vi "MTExam.vi"() -> ()   [LabVIEW 2016]
uses:
  VIs/uPythonX/uPythonX.xctl
panel:
  in  "WiFi":T1(xcontrol)={"VISA Refnum in"="ASRL44::INSTR", "Python Code"="import machine, network, ubinascii, ujson, urequests, utime,gc\nfrom pyb import LED\n\nWiFi = network.WLAN()\n\nmac = ubinascii.hexlify(network.WLAN().config(\"mac\"),\":\").decode()\nprint(\"MAC address: \" + mac)\ndef connect():\n     if not WiFi.isconnected():\n          print (\"Connecting ..\")\n          WiFi.active(True)\n          WiFi.connect(\"Rogers\",\"s0meth1ng\")\n          i=0\n          while i < 25 and not WiFi.isconnected():\n               utime.sleep_ms(200)\n               i=i+1\n          if WiFi.isconnected():\n               print (\"Connection succeeded\")\n          else:\n               print (\"Connection failed\")     \n     return WiFi.isconnected()\n\n# Systemlink\nKey = \"dYy-vDU9TXxDCy2QG3jO4J0s1-QUyYs6sO1xPd1oKQ\"\n\nurlBase = \"https://api.systemlinkcloud.com/nitag/v2/tags/\"\n\nheaders = {\"Accept\":\"application/json\",\"x-ni-api-key\":Key}\n\ndef Put(tag,type,value):\n     urlTag = urlBase + tag\n     urlValue = urlBase + tag + \"/values/current\"\n     propName={\"type\":type,\"path\":tag}\n     propValue = {\"value\":{\"type\":type,\"value\":value}}\n     #  assume that the tag is already created  -      urequests.put(urlTag,headers=headers,json=propName).text\n     try:\n          response = urequests.put(urlValue,headers=headers,json=propValue)\n          print(response.text)\n          response.close()\n     except:\n          print('error')\n\ndef Get(tag):\n     urlValue = urlBase + tag + \"/values/current\"\n     try:\n          response = urequests.get(urlValue,headers=headers)\n          value = response.text\n          response.close()\n          print(value)\n          data = ujson.loads(value)\n          result = data.get(\"value\").get(\"value\")\n     except:\n          print('error')\n          result = 'error'\n     return result\n\nprint (\"WiFi: \",connect())\nPut('EV3','U_INT64','3')\nGet('EV3')\nGet('msec')\nPut('msec','INT',100)\nled = LED(1) # 1=red, 2=green, 3=blue\n\ni=0\nold = utime.ticks_ms()\nwhile True:\n     Put('EV3','U_INT64',str(i))\n     new = utime.ticks_ms()\n     Put('msec','INT',str(new-old))\n     old = new\n     i= i + 1\n     print(i)\n     led.toggle()\n     utime.sleep_ms(20)\n     gc.collect()\n\n\n\n\n\n\n"}
  in  "PyBoard - Tacho":T1(xcontrol)={"VISA Refnum in"="ASRL44::INSTR", "Python Code"="# From https://github.com/peterhinch/micropython-samples/blob/master/encoders/encoder.py\n\nfrom pyb import Pin\nimport utime\nfrom machine import UART\n\nuart = UART(3)  #TX = Y9\nuart.init(9600, bits=8, parity=None, stop=1)\n\nclass Encoder(object):\n     def __init__(self, pin_x, pin_y, reverse, scale):\n          self.reverse = reverse\n          self.scale = scale\n          self.forward = True\n          self.pin_x = pin_x\n          self.pin_y = pin_y\n          self._pos = 0\n          self.x_interrupt = pyb.ExtInt(pin_x, pyb.ExtInt.IRQ_RISING_FALLING, pyb.Pin.PULL_NONE, self.x_callback)\n          self.y_interrupt = pyb.ExtInt(pin_y, pyb.ExtInt.IRQ_RISING_FALLING, pyb.Pin.PULL_NONE, self.y_callback)\n\n     def x_callback(self, line):\n          self.forward = self.pin_x.value() ^ self.pin_y.value() ^ self.reverse\n          self._pos += 1 if self.forward else -1\n\n     def y_callback(self, line):\n          self.forward = self.pin_x.value() ^ self.pin_y.value() ^ self.reverse ^ 1\n          self._pos += 1 if self.forward else -1\n\n     @property\n     def position(self):\n          return self._pos*self.scale\n\n     def reset(self):\n          self._pos = 0\n\npin1 = Pin('Y4', Pin.IN)\npin2 = Pin('Y3', Pin.IN)\n\ne=Encoder(pin1,pin2,False,0.5)\ne.reset()\nwhile True:\n     value = e.position\n     sent = uart.write('%d\\n' % int(value/10))\n     print(value)\n     utime.sleep(1)\n\n\n\n\n"}
  in  "Trinket":T1(xcontrol)={"VISA Refnum in"="ASRL47::INSTR", "Python Code"="'''\nhttps://circuitpython.readthedocs.io/en/2.x/shared-bindings/busio/UART.html\n     \nconnect D3 and D4 to test\n'''\n\nimport board\nfrom busio import UART\nimport adafruit_dotstar as dotstar\n\nuart=UART(board.D4,board.D3,timeout=2000) # tx, rx\ndot = dotstar.DotStar(board.APA102_SCK, board.APA102_MOSI, 1, brightness=0.2)\n\n\nuart.write('test')\nuart.read(4)\n\nuart.write('2\\n')\n\nwhile True:\n     value = uart.readline()\n     print(value)\n     if value:\n          dot[0] = int(value)\n\n\n\n\n\n\n\n"}
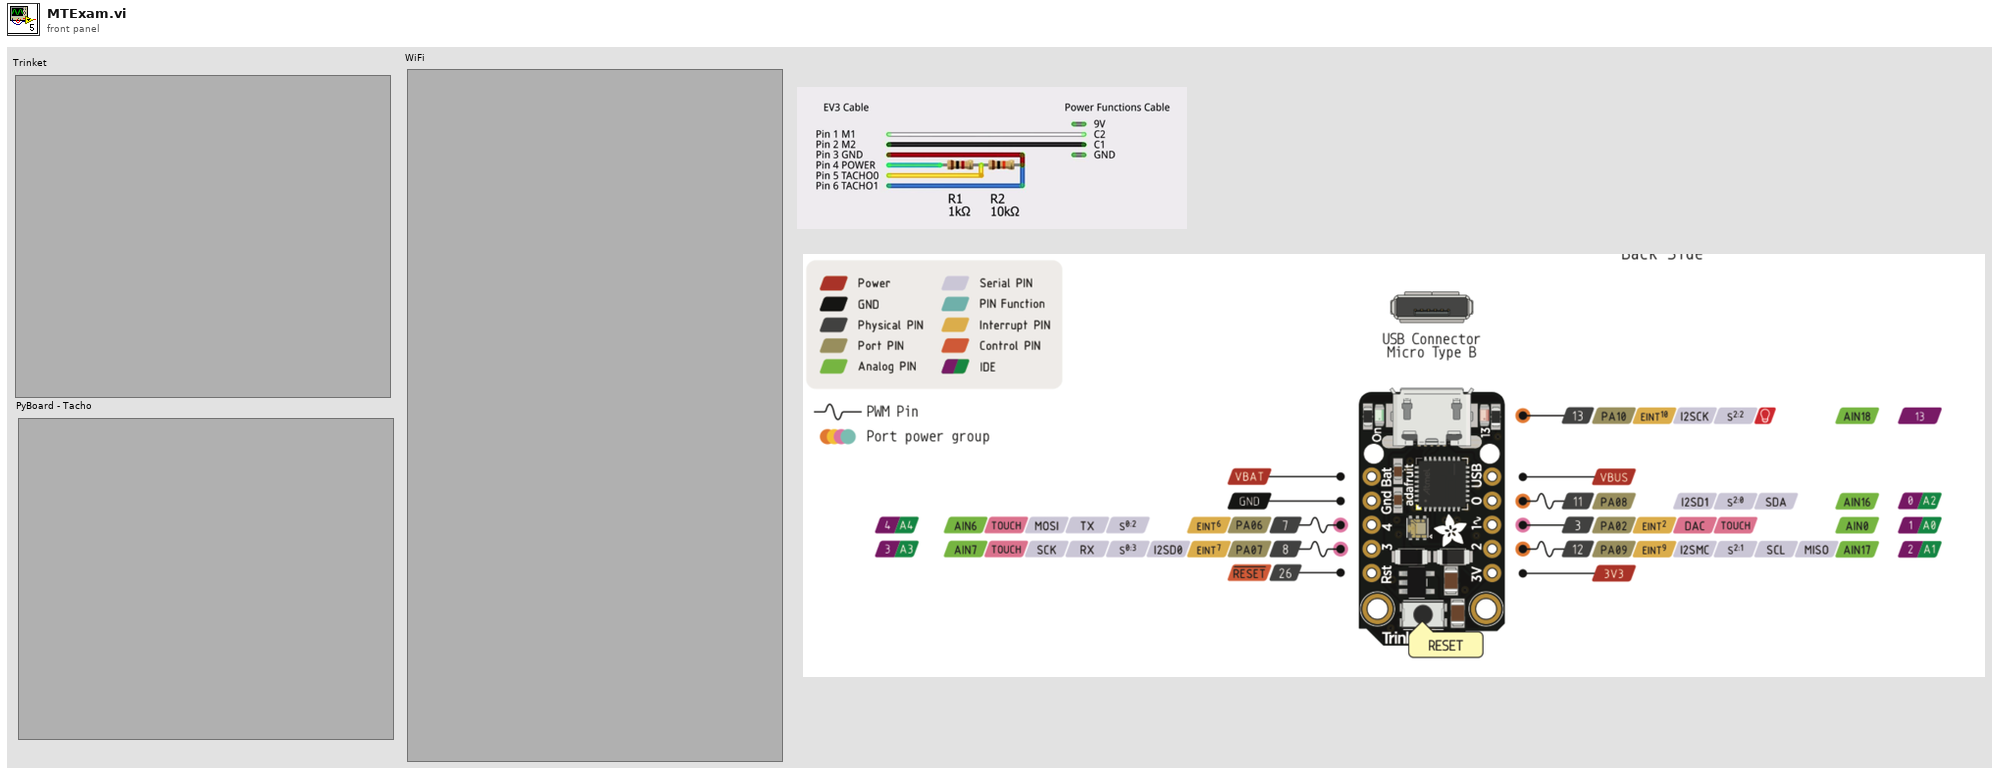
[diagram p1: front panel]
types:
  T1 = cluster{"VISA Refnum in":refnum<visa-resource-name>, "Python Code":string}
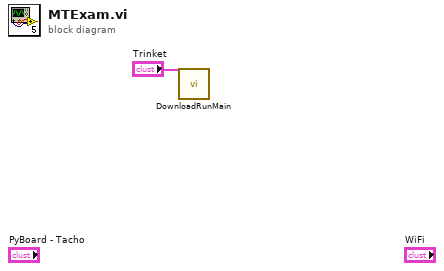
[diagram p0: block diagram]
diagram:
  n1 = call "DownloadRunMain.vi"("Data In"="Trinket") -> ()  [unwired: 8 in, 3 out]
